vi "SimulateTerminalVoltage.vi"() -> (3 "Simulated Terminal Voltage":dbl[][](array[numeric])=[[0.1]])   [LabVIEW 2012]
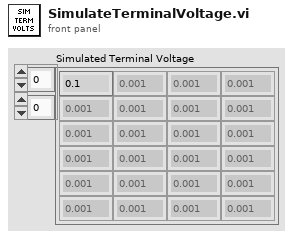
[diagram p1: front panel]
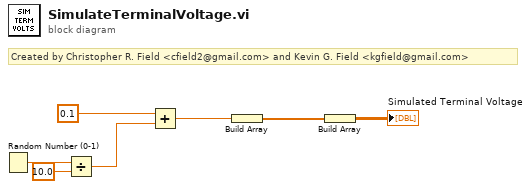
[diagram p0: block diagram]
diagram:
  # "Created by Christopher R. Field <cfield2@gmail.com> and Kevin G. Field <kgfield@gmail.com>"
  n1 = Random Number (0-1)() -> (number: 0 to 1=w7:dbl)
  n2 = Divide(x=w7, y=10.0) -> (x/y=w4:dbl)
  n3 = Add(x=0.1, y=w4) -> (x+y=w3:dbl)
  n4 = Build Array(w3) -> (w2:dbl[])
  n5 = Build Array(w2) -> (→"Simulated Terminal Voltage":dbl[][])
